vi "Move Piezo.vi"(8 "error in (no error)":errorcluster, 10 "Move to (um)":sgl, 11 "Hardware Resources In":T1={"Piezo Serial Number"=41848555, "MG17Piezo"=refnum, "Setpoint (um)"=0.0}) -> (0 "error out":errorcluster, 3 "Hardware Resources Out":T1={"Piezo Serial Number"=41848555, "MG17Piezo"=refnum, "Setpoint (um)"=0.0})   [LabVIEW 2013]
uses:
  Hardware Configuration.ctl
  Piezo.lvlib
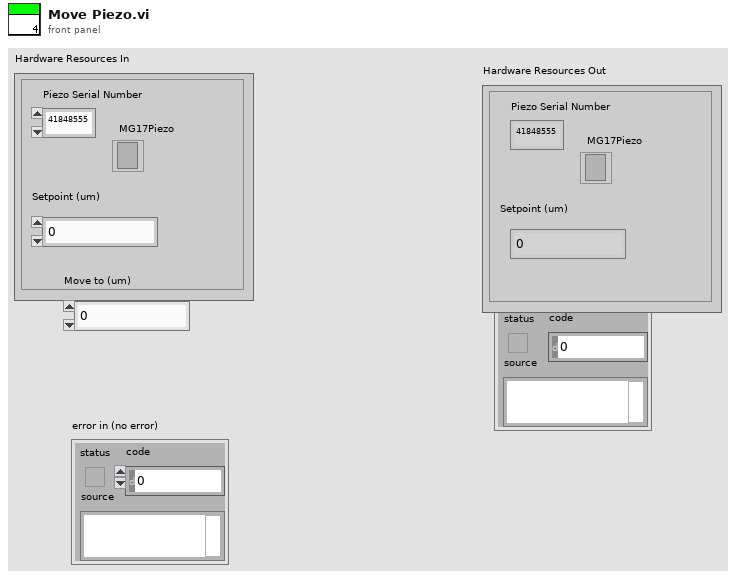
[diagram p1: front panel]
types:
  T1 = typedef "Piezo.lvlib/Hardware Configuration.ctl" = cluster{"Piezo Serial Number":i32, "MG17Piezo":refnum<k7>, "Setpoint (um)":sgl}
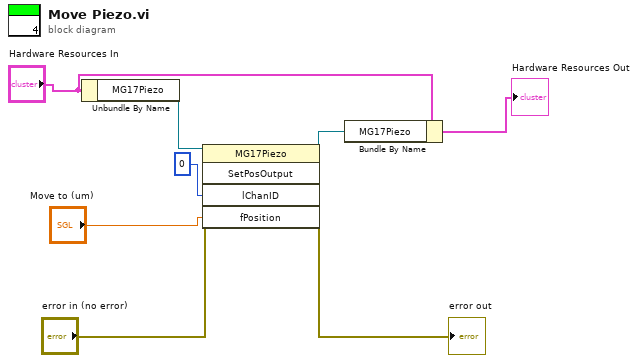
[diagram p0: block diagram]
diagram:
  n1 = Unbundle By Name("Hardware Resources In") -> ("MG17Piezo"=w6:refnum<k7>)
  n2 = invoke class="MG17Piezo" method="SetPosOutput"(reference=w6, error in="error in (no error)", "lChanID"=0, "fPosition"="Move to (um)") -> (reference out=w1:refnum<k7>, error out=→"error out":errorcluster)  [unwired: 1 in, 3 out]
  n3 = Bundle By Name(cluster="Hardware Resources In", "MG17Piezo"=w1) -> (→"Hardware Resources Out":T1)
